vi "Unflatten (offset).vi"(8 "error in (no error)":errorcluster, 9 "offset (0)":i32, 10 "JSON stream":string, 11 "JSON Array in":refnum<class "JSON Array.lvclass">) -> (0 "error out":errorcluster, 1 "offset":i32, 3 "JSON Array out":refnum<class "JSON Array.lvclass">, 4 "Empty?":bool)   [LabVIEW 2011, in "JSON Array.lvclass"]
uses:
  JSON Array.lvclass
  JSON Value/JSON Value.lvclass
  JSON Array.lvclass/JSON Array.ctl
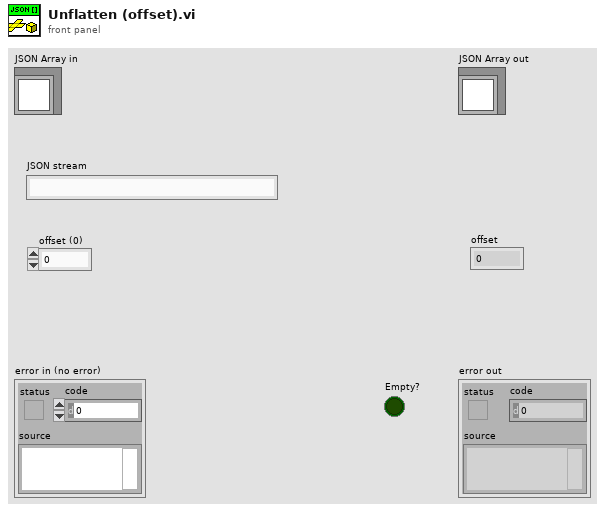
[diagram p1: front panel]
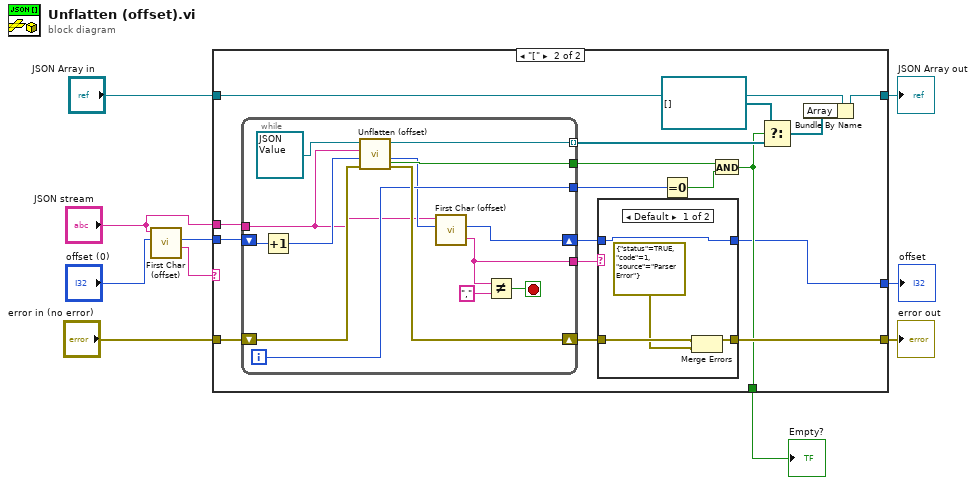
[diagram p0: block diagram]
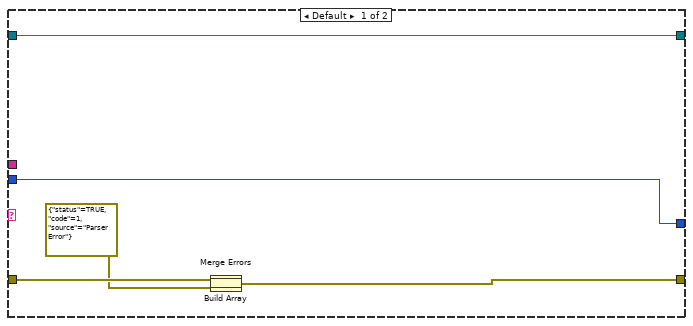
[diagram p2: hidden frame]
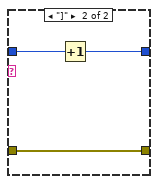
[diagram p3: hidden frame]
diagram:
  n1 = call "First Char (offset).vi"("offset (0)"="offset (0)", "String in"="JSON stream") -> ("First Char"=w4:string, "Offset"=w3:i32)  [unwired: 8 in]
  n2 = case shown="\"[\"" w4 {
    tunnel: "JSON stream" -> [_ w33]
    tunnel: [w15 w28] -> w10
    tunnel: "error in (no error)" -> [w16 w30]
    tunnel: [w13 w31] -> w8
    tunnel: "JSON Array in" -> [w13 w32]
    tunnel: [_ w20] -> w6
    tunnel: w3 -> [w11 w19]
    tunnel: [w11 w17] -> w2
    frame Default {
      n3 = Build Array(w16, errorcluster {"status"=TRUE, "code"=1, "source"="Parser Error"} ("error in")) -> (w12:errorcluster[])
      n4 = Merge Errors(w12) -> (w15:errorcluster)
    }
    frame "[" {
      n5 = while {
        tunnel: [w52] -> w22 mode=indexing
        tunnel: [w51] -> w29
        shift-right: [w49] -> w27
        shift-left: w30 -> [w50]
        tunnel: [w47] -> w25
        tunnel: [w46] -> w24
        shift-right: [w42] -> w18
        shift-left: w19 -> [w45]
        tunnel: w33 -> [w41]
        i -> [w46]
        stop <- w53 stop-if-true
        n6 = Increment(x=w45) -> (x+1=w44:i32)
        n7 = call-dynamic "Unflatten (offset).vi"("error in (no error)"=w50, "offset (0)"=w44, "JSON stream"=w41, "JSON Value in"=refnum<class "JSON Value.lvclass"> refnum ("JSON Value.lvclass")) -> ("error out"=w49:errorcluster, "offset"=w43:i32, "JSON Value out"=w52:refnum<class "JSON Value.lvclass">, "Empty?"=w47:bool)  [unwired: 4 in]
        n8 = call "First Char (offset).vi"("offset (0)"=w43, "String in"=w41) -> ("First Char"=w51:string, "Offset"=w42:i32)  [unwired: 8 in]
        n9 = Not Equal?(x=w51, y=",") -> (x != y?=w53:bool)
      }
      n10 = case shown="Default" w29 {
        tunnel: [w37 w40] -> w28
        tunnel: w27 -> [w36 w40]
        tunnel: w18 -> [w34 w39]
        tunnel: [w34 w38] -> w17
        frame Default {
          n11 = Merge Errors(w36, errorcluster {"status"=TRUE, "code"=1, "source"="Parser Error"} ("error in")) -> (w37:errorcluster)
        }
        frame "]" {
          n12 = Increment(x=w39) -> (x+1=w38:i32)
        }
      }
      n13 = Equal To 0?(x=w24) -> (x = 0?=w26:bool)
      n14 = And(x=w25, y=w26) -> (x .and. y?=w20:bool)
      n15 = Select(t=refnum<class "JSON Value.lvclass">[] [], s=w20, f=w22) -> (s? t:f=w23:refnum<class "JSON Value.lvclass">[])
      n16 = Bundle By Name(cluster=w32, "Array"=w23) -> (w31:refnum<class "JSON Array.lvclass">)
    }
  }
  "error out" <- w10
  "JSON Array out" <- w8
  "Empty?" <- w6
  "offset" <- w2
